vi "AssertGreaterThan_Tests.vi"() -> (15 "error out":errorcluster)   [LabVIEW 2016, in "DronaTest.lvlib"]
uses:
  DronaTest.lvlib
  APIs/Assert/AssertControlValue/Greater.vi
  <vilib>/addons/_JKI Toolkits/Caraya/classes/Assert/Assert Greater_Variant.vi
  <vilib>/addons/_JKI Toolkits/Caraya/classes/Assert/Assert Error.vi
  APIs/Assert/AssertControlValue/GreaterOrEqual.vi
  <vilib>/addons/_JKI Toolkits/Caraya/classes/Assert/Assert Greater Or Equal_Variant.vi
  <vilib>/addons/_JKI Toolkits/Caraya/classes/Test/Test.lvclass
  Drona.lvlib
  <vilib>/addons/_JKI Toolkits/Caraya/classes/Assert/Assert.lvclass
  APIs/Assert/AssertControlValue/AssertControlValue.lvlib
panel:
  in  "error in":errorcluster
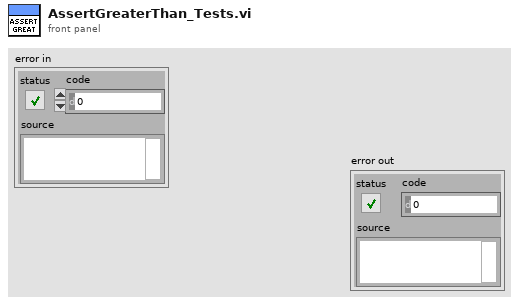
[diagram p1: front panel]
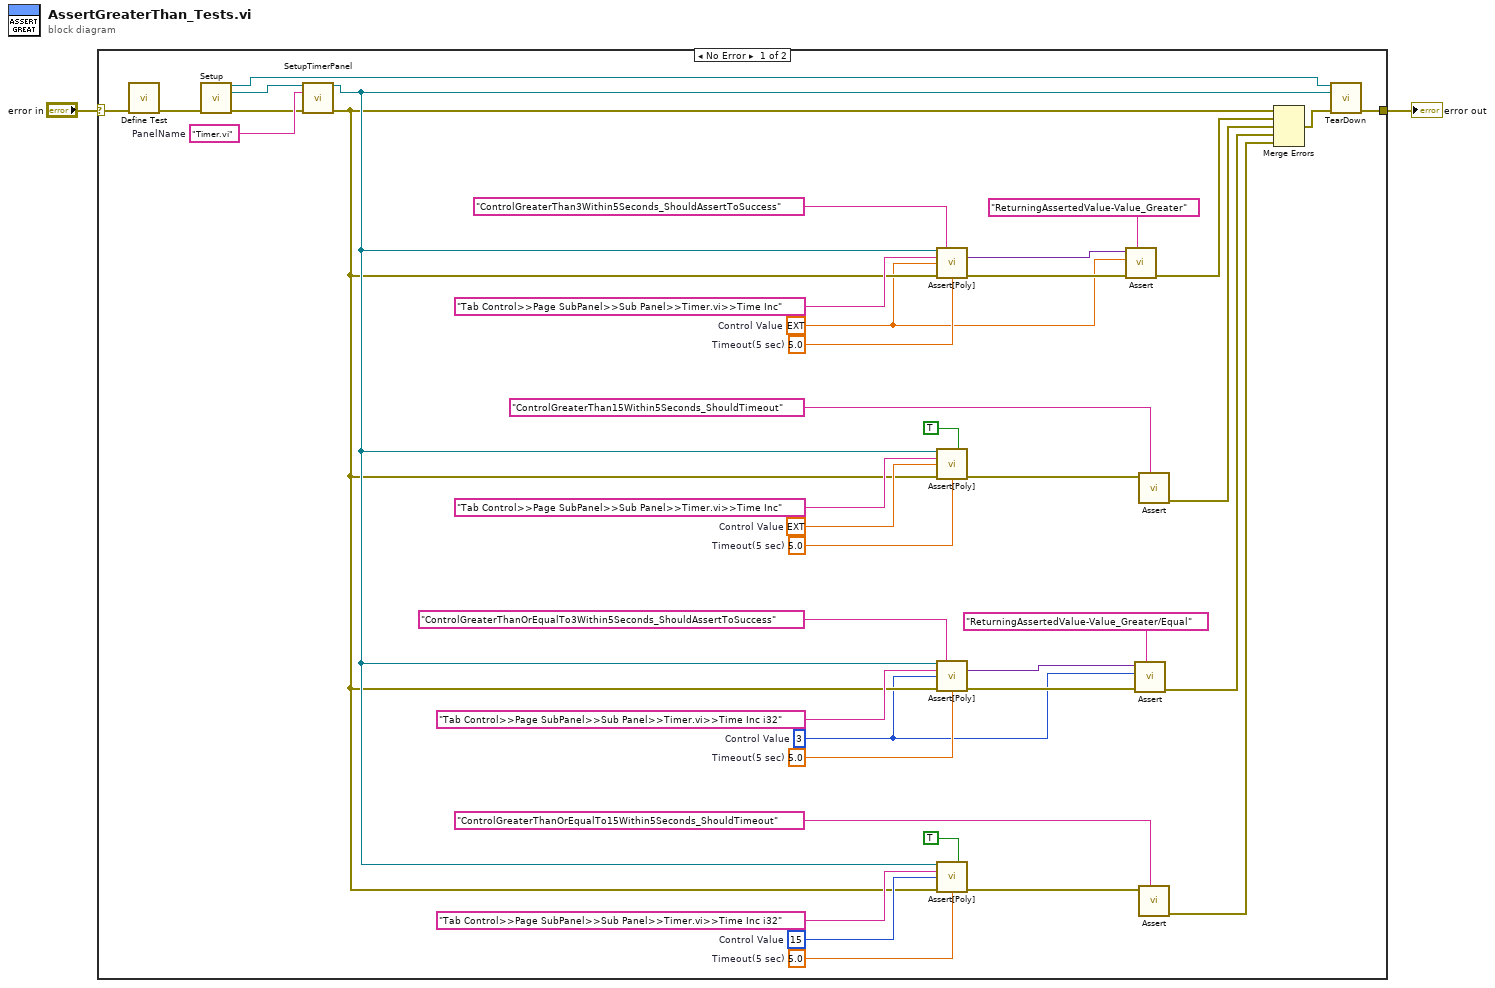
[diagram p0: block diagram]
diagram:
  n1 = case shown="No Error" "error in" {
    selector: "error in" -> [w42 w43]
    tunnel: [w17 w43] -> w1
    frame No Error {
      w23 = "Timer.vi"  # PanelName
      w31 = 5.0  # Timeout(5 sec)
      w5 = 3  # Control Value
      w30 = 5.0  # Timeout(5 sec)
      w29 = 15  # Control Value
      w34 = 5.0  # Timeout(5 sec)
      w3 = ext 3.0  # Control Value
      w35 = 5.0  # Timeout(5 sec)
      w36 = ext 15.0  # Control Value
      n2 = call <vilib>:"Define Test.vi"("error in (no error)"=w42) -> ("error out"=w20:errorcluster)  [unwired: 9 in, 1 out]
      n3 = call "Setup.vi"("error in (no error)"=w20) -> ("Application Ref"=w19:refnum<vi>, "VI out"=w21:refnum<vi>, "error out"=w22:errorcluster)  [unwired: 12 in]
      n4 = call "SetupTimerPanel.vi"("VI in"=w21, "Item Name"=w23, "error in (no error)"=w22) -> ("VI out"=w16:refnum<vi>, "error out"=w15:errorcluster)  [unwired: 11 in]
      n5 = call-poly "Assert[Poly].vi"("VI Reference In"=w16, "Test Label"="ControlGreaterThan3Within5Seconds_ShouldAssertToSuccess" ("string"), "Control Path"="Tab Control>>Page SubPanel>>Sub Panel>>Timer.vi>>Time Inc", "Control Value"=w3, "Error In"=w15, "Timeout(5 sec)"=w34) -> ("Asserted Value"=w4:variant, "Error Out"=w12:errorcluster)  [unwired: 7 in, 1 out]
      n6 = call-poly "Assert[Poly].vi"("VI Reference In"=w16, "Assert Only? (F)"=TRUE, "Control Path"="Tab Control>>Page SubPanel>>Sub Panel>>Timer.vi>>Time Inc", "Control Value"=w36, "Error In"=w15, "Timeout(5 sec)"=w35) -> ("Error Out"=w38:errorcluster)  [unwired: 7 in, 2 out]
      n7 = call-poly "Assert[Poly].vi"("VI Reference In"=w16, "Test Label"="ControlGreaterThanOrEqualTo3Within5Seconds_ShouldAssertToSuccess" ("string"), "Control Path"="Tab Control>>Page SubPanel>>Sub Panel>>Timer.vi>>Time Inc i32", "Control Value"=w5, "Error In"=w15, "Timeout(5 sec)"=w31) -> ("Asserted Value"=w6:variant, "Error Out"=w9:errorcluster)  [unwired: 7 in, 1 out]
      n8 = call-poly "Assert[Poly].vi"("VI Reference In"=w16, "Assert Only? (F)"=TRUE, "Control Path"="Tab Control>>Page SubPanel>>Sub Panel>>Timer.vi>>Time Inc i32", "Control Value"=w29, "Error In"=w15, "Timeout(5 sec)"=w30) -> ("Error Out"=w27:errorcluster)  [unwired: 7 in, 2 out]
      n9 = call-poly <vilib>:"Assert.vi"("Label"="ReturningAssertedValue-Value_Greater", "error in (no error)"=w12, "Y"=w3, "X"=w4) -> ("error out"=w11:errorcluster)  [unwired: 6 in, 1 out]
      n10 = call-poly <vilib>:"Assert.vi"("Label"="ReturningAssertedValue-Value_Greater/Equal", "error in (no error)"=w9, "Y"=w5, "X"=w6) -> ("error out"=w8:errorcluster)  [unwired: 6 in, 1 out]
      n11 = call-poly <vilib>:"Assert.vi"("Label"="ControlGreaterThan15Within5Seconds_ShouldTimeout" ("string"), "Error?"=w38) -> ("error out"=w41:errorcluster)  [unwired: 8 in, 1 out]
      n12 = call-poly <vilib>:"Assert.vi"("Label"="ControlGreaterThanOrEqualTo15Within5Seconds_ShouldTimeout" ("string"), "Error?"=w27) -> ("error out"=w24:errorcluster)  [unwired: 8 in, 1 out]
      n13 = Merge Errors(w15, w11, w41, w8, w24) -> (w18:errorcluster)
      n14 = call "TearDown.vi"("Application Ref"=w19, "VI in"=w16, "error in (no error)"=w18) -> ("error out"=w17:errorcluster)  [unwired: 12 in]
    }
    frame Error {
    }
  }
  "error out" <- w1
